vi "Test_Remove.vi"(8 "error in (no error)":errorcluster, 11 "TestCase in":refnum<class "StringList_Delegations.lvclass">) -> (0 "error out":errorcluster, 3 "TestCase out":refnum<class "StringList_Delegations.lvclass">)   [LabVIEW 2009, in "StringList_Delegations.lvclass"]
uses:
  StringList_Delegations.lvclass
  StringList_Delegations.lvclass/StringList_Delegations.ctl
  source/Lists.Interfaces/StringList/StringList.lvclass
  Test Doubles/ListImp_RefSpy/ListImp_RefSpy.lvclass
  UnitTestComparisons/UnitTestComparisons.lvlib
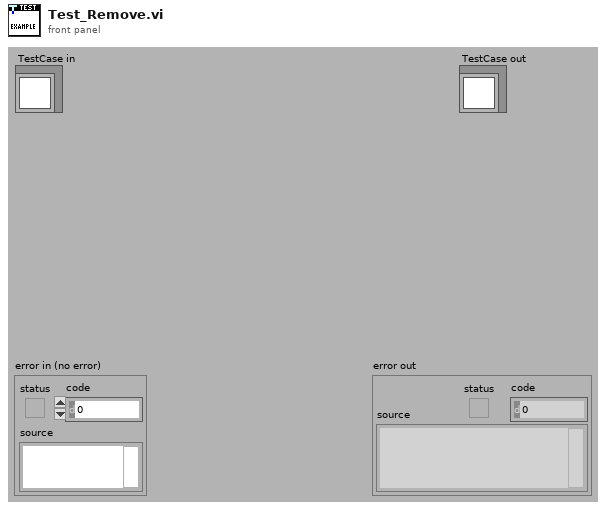
[diagram p1: front panel]
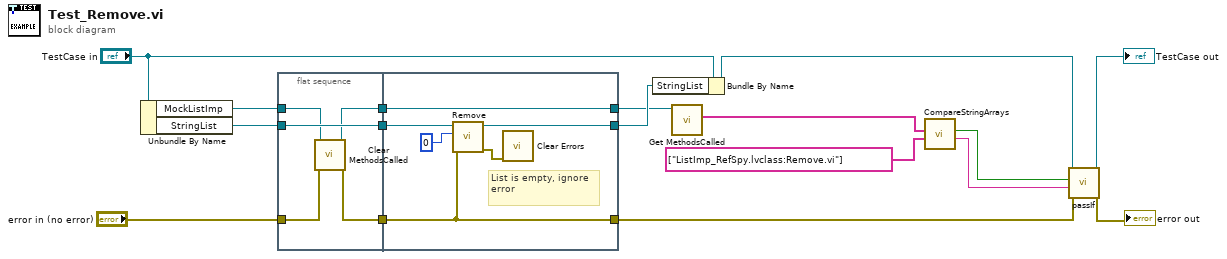
[diagram p0: block diagram]
diagram:
  n1 = Unbundle By Name("TestCase in") -> ("MockListImp"=w12:refnum<class "ListImp_RefSpy.lvclass">, "StringList"=w14:refnum<class "StringList.lvclass">)
  n2 = flat-sequence {
    tunnel: w12 -> [w21]
    tunnel: "error in (no error)" -> [w19]
    tunnel: w14 -> [w22]
    tunnel: [w22] -> w11
    tunnel: [w18] -> w10
    tunnel: [w20] -> w9
    tunnel: w11 -> [w28]
    tunnel: w10 -> [w24]
    tunnel: w9 -> [w26]
    tunnel: [w24] -> w5
    tunnel: [w27] -> w7
    tunnel: [w26] -> w6
    frame #0 {
      n3 = call "Clear MethodsCalled.vi"("error in (no error)"=w19, "MockListImp in"=w21) -> ("error out"=w18:errorcluster, "MockListImp out"=w20:refnum<class "ListImp_RefSpy.lvclass">)  [unwired: 8 in]
    }
    frame #1 {
      # "List is empty, ignore error"
      n4 = call-dynamic "Remove.vi"("error in (no error)"=w24, "Index"=0, "StringList in"=w28) -> ("error out"=w23:errorcluster, "StringList out"=w27:refnum<class "StringList.lvclass">)  [unwired: 6 in, 1 out]
      n5 = call <vilib>:"Clear Errors.vi"("error in (no error)"=w23) -> ()  [unwired: 6 in, 1 out]
    }
  }
  n6 = Bundle By Name(cluster="TestCase in", "StringList"=w7) -> (w8:refnum<class "StringList_Delegations.lvclass">)
  n7 = call "Get MethodsCalled.vi"("MockListImp"=w6) -> ("MethodsCalled"=w4:string[])  [unwired: 9 in, 1 out]
  n8 = call "CompareStringArrays.vi"("Expected Strings"=string[] ["ListImp_RefSpy.lvclass:Remove.vi"] ("MethodsCalled"), "Actual Strings"=w4) -> ("Message"=w1:string, "Equal?"=w2:bool)  [unwired: 8 in]
  n9 = call-dynamic "passIf.vi"("error in (no error)"=w5, "message (\"\")"=w1, "pass"=w2, "TestCase in"=w8) -> ("error out"=→"error out":errorcluster, "TestCase out"=→"TestCase out":refnum<class "StringList_Delegations.lvclass">)  [unwired: 6 in]
